vi "hw2p4_hickey.vi"() -> ()   [LabVIEW 2014]
panel:
  in  "stop":bool
  in  "Beeps Per Minute":dbl
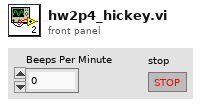
[diagram p1: front panel]
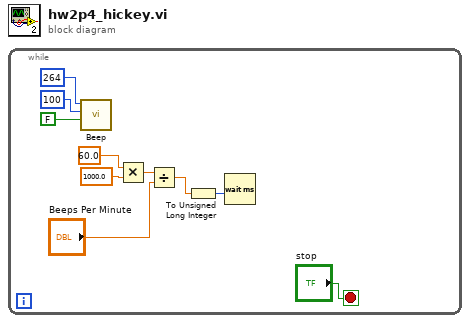
[diagram p0: block diagram]
diagram:
  n1 = while {
    stop <- "stop" stop-if-true
    n2 = call <vilib>:"Beep.vi"("use system alert? (T)"=FALSE, "duration (msec)"=u32 100, "frequency (Hz)"=u32 264) -> ()  [unwired: 9 in]
    n3 = Multiply(x=60.0, y=1000.0) -> (x*y=w3:dbl)
    n4 = Divide(x=w3, y="Beeps Per Minute") -> (x/y=w2:dbl)
    n5 = To Unsigned Long Integer(number=w2) -> (unsigned 32bit integer=w1:u32)
    n6 = Wait (ms)(milliseconds to wait=w1) -> ()  [unwired: 1 out]
  }
